vi "Helper Objects bottom cords.vi"(2 "error in (no error)":errorcluster, 3 "Rectangle":T2 {"Rotation" format="%.2f"; "Left" scale=0.0..1024.0; "Right" scale=0.0..1024.0; "Bottom" scale=1024.0..0.0; "Top" scale=1024.0..0.0}, 4 "Object color":dbl, 5 "Image matrix":T1) -> (0 "error out":errorcluster, 1 "Objects Bottom Cords":cluster{"X":dbl, "Y":dbl, "Angle":dbl}[](array[cluster]))   [LabVIEW 2009, in "ImageAnalysis.lvlib"]
doc: "Input:\n- A image represented as a matrix. (The image should be the output of the IMAQ Label function).s\n- The color to look for.\n- The region to look in.\n\nOutput:\n- A 1-D array with the objects bottom cordinates."
uses:
  ImageAnalysis.lvlib
  <vilib>/Analysis/Matrix/Datatypes/RealMatrix.ctl
  <vilib>/Analysis/Matrix/NI_Matrix.lvlib
panel:
  in  "Point":cluster{"X":dbl, "Y":dbl, "Angle":dbl}
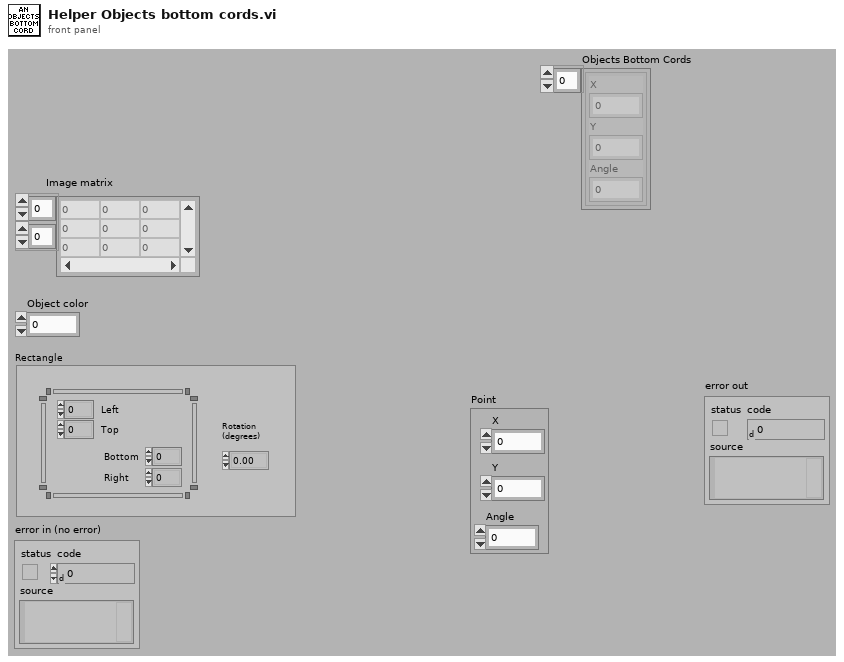
[diagram p1: front panel]
types:
  T1 = typedef "NI_Matrix.lvlib/RealMatrix.ctl" = dbl[][]
  T2 = typedef "IMAQ Rectangle" = cluster{"Left":i32, "Top":i32, "Right":i32, "Bottom":i32, "Rotation":dbl}
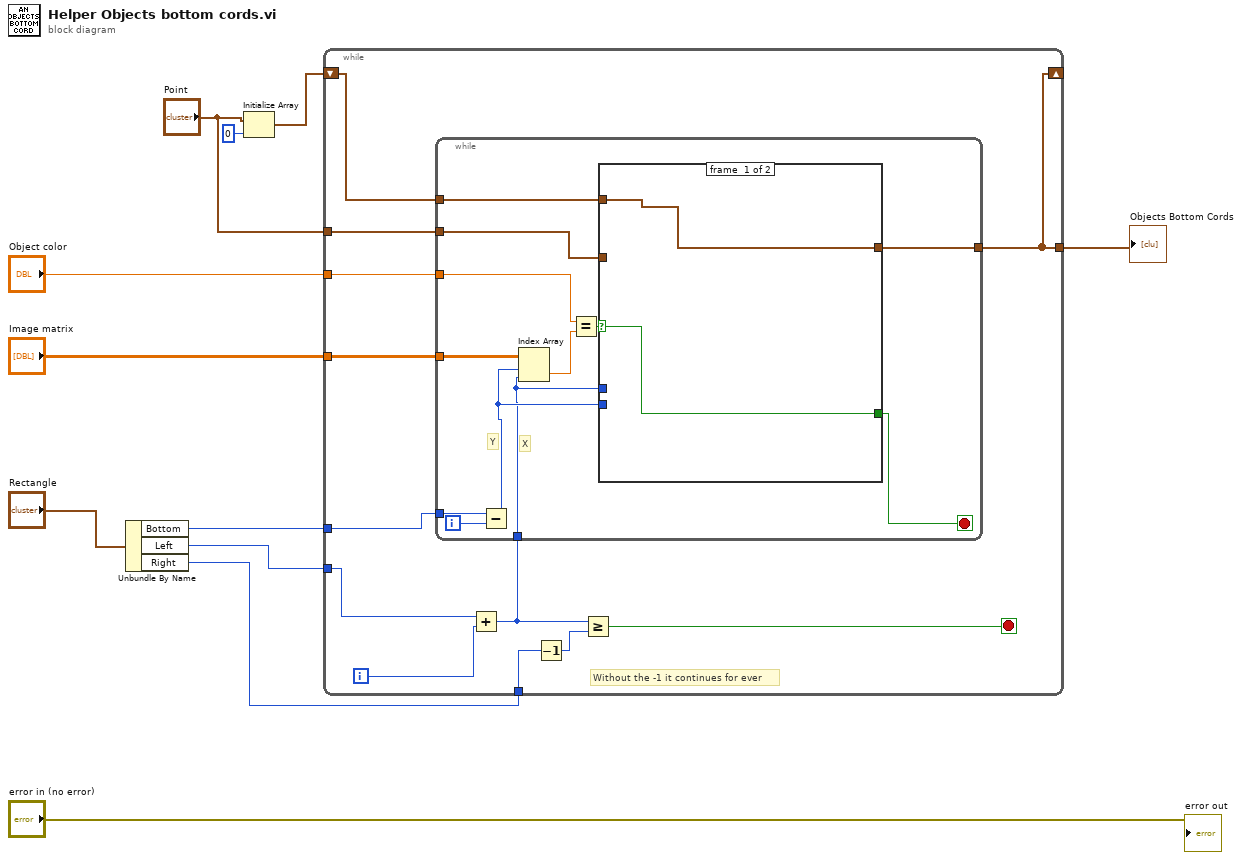
[diagram p0: block diagram]
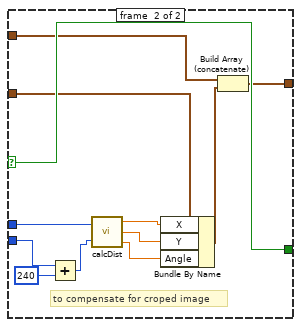
[diagram p2: hidden frame]
diagram:
  n1 = Unbundle By Name("Rectangle") -> ("Bottom"=w8:i32, "Left"=w9:i32, "Right"=w10:i32)
  n2 = Initialize Array("Point", 0 ("dimension size")) -> (w2:cluster{"X":dbl, "Y":dbl, "Angle":dbl}[])
  n3 = while {
    tunnel: w9 -> [w20]
    tunnel: w10 -> [w17]
    tunnel: w8 -> [w23]
    tunnel: "Image matrix" -> [w22]
    tunnel: "Object color" -> [w21]
    tunnel: [w13] -> w5
    shift-right: [w13] -> _
    shift-left: w2 -> [w14]
    tunnel: "Point" -> [w12]
    i -> [w15]
    stop <- w18 stop-if-true
    # "Without the -1 it continues for ever"
    n4 = Add(x=w20, y=w15) -> (x+y=w19:i32)
    n5 = while {
      tunnel: w23 -> [w35]
      tunnel: w22 -> [w27]
      tunnel: w21 -> [w30]
      tunnel: w19 -> [w24]
      tunnel: w14 -> [w29]
      tunnel: [w28] -> w13
      tunnel: w12 -> [w26]
      i -> [w34]
      stop <- w33 stop-if-true
      # "X"
      # "Y"
      n6 = Subtract(x=w35, y=w34) -> (x-y=w25:i32)
      n7 = Index Array(array=w27, index (row)=w25, index (col)=w24) -> (element=w31:dbl)
      n8 = Equal? ("Equal.vi")(x=w30, y=w31) -> (x = y?=w32:bool)
      n9 = case shown="True" w32 {
        selector: w32 -> [w37 w49]
        tunnel: [w37 w49] -> w33
        tunnel: w29 -> [w36 w47]
        tunnel: [w36 w48] -> w28
        tunnel: w26 -> [_ w45]
        tunnel: w25 -> [_ w40]
        tunnel: w24 -> [_ w44]
        frame #0 {
        }
        frame #1 {
          # "to compensate for croped image"
          n10 = Add(x=w40, y=240) -> (x+y=w39:i32)
          n11 = call "calcDist.vi"("X-cord"=w44, "Y-cord"=w39) -> ("Distance sideways to pixel"=w43:dbl, "Distance to pixel"=w42:dbl, "Angle to pixel"=w41:dbl)
          n12 = Bundle By Name(cluster=w45, "X"=w43, "Y"=w42, "Angle"=w41) -> (w46:cluster{"X":dbl, "Y":dbl, "Angle":dbl})
          n13 = Build Array (concatenate)(w47, w46) -> (w48:cluster{"X":dbl, "Y":dbl, "Angle":dbl}[])
        }
      }
    }
    n14 = Decrement(x=w17) -> (x-1=w16:i32)
    n15 = Greater Or Equal?(x=w19, y=w16) -> (x >= y?=w18:bool)
  }
  "Objects Bottom Cords" <- w5
  "error out" <- "error in (no error)"
